vi "GeoData.vi"() -> ()   [LabVIEW 2017] (continued)
63130\t29189\tSaint louis\tMO\tSt. Louis County\tH1\n63133\t29189\tSaint louis\tMO\tSt. Louis County\tH1\n63138\t29189\tSaint louis\tMO\tSt. Louis County\tH1\n63011\t29189\tBallwin\tMO\tSt. Louis County\tH1\n63006\t29189\tChesterfield\tMO\tSt. Louis County\tH1\n63042\t29189\tHazelwood\tMO\tSt. Louis County\tH1\n63141\t29189\tSaint louis\tMO\tSt. Louis County\tH1\n63140\t29189\tSaint louis\tMO\tSt. Louis County\tH1\n63021\t29189\tBallwin\tMO\tSt. Louis County\tH1\n63117\t29189\tSaint louis\tMO\tSt. Louis County\tH1\n63121\t29189\tSaint louis\tMO\tSt. Louis County\tH1\n63126\t29189\tSaint louis\tMO\tSt. Louis County\tH1\n63025\t29189\tEureka\tMO\tSt. Louis County\tH1\n63022\t29189\tBallwin\tMO\tSt. Louis County\tH1\n63045\t29189\tEarth city\tMO\tSt. Louis County\tH1\n63167\t29189\tSaint louis\tMO\tSt. Louis County\tH1\n65340\t29195\tMarshall\tMO\tSaline County\tH1\n65349\t29195\tSlater\tMO\tSaline County\tH1\n64020\t29195\tConcordia\tMO\tSaline County\tH1\n65351\t29195\tSweet springs\tMO\tSaline County\tH1\n65339\t29195\tMalta bend\tMO\tSaline County\tH1\n65344\t29195\tMiami\tMO\tSaline County\tH1\n65322\t29195\tBlackwater\tMO\tSaline County\tH1\n65347\t29195\tNelson\tMO\tSaline County\tH1\n65320\t29195\tArrow rock\tMO\tSaline County\tH1\n65333\t29195\tHoustonia\tMO\tSaline County\tH1\n64096\t29195\tWaverly\tMO\tSaline County\tH1\n65330\t29195\tGilliam\tMO\tSaline County\tH1\n65327\t29195\tEmma\tMO\tSaline County\tH1\n65321\t29195\tBlackburn\tMO\tSaline County\tH1\n63535\t29197\tCoatsville\tMO\tSchuyler County\tH1\n63548\t29197\tLancaster\tMO\tSchuyler County\tH1\n63536\t29197\tDowning\tMO\tSchuyler County\tH1\n63541\t29197\tGlenwood\tMO\tSchuyler County\tH1\n63561\t29197\tQueen city\tMO\tSchuyler County\tH1\n63546\t29197\tGreentop\tMO\tSchuyler County\tH1\n63543\t29199\tGorin\tMO\tScotland County\tH1\n63555\t29199\tMemphis\tMO\tScotland County\tH1\n63563\t29199\tRutledge\tMO\tScotland County\tH1\n63442\t29199\tGranger\tMO\tScotland County\tH1\n63432\t29199\tArbela\tMO\tScotland County\tH1\n63735\t29201\tBell city\tMO\tScott County\tH1\n63742\t29201\tCommerce\tMO\tScott County\tH1\n63758\t29201\tKelso\tMO\tScott County\tH1\n63774\t29201\tPerkins\tMO\tScott County\tH1\n63771\t29201\tOran\tMO\tScott County\tH1\n63740\t29201\tChaffee\tMO\tScott County\tH1\n63834\t29201\tCharleston\tMO\tScott County\tH1\n63780\t29201\tScott city\tMO\tScott County\tH1\n63801\t29201\tSikeston\tMO\tScott County\tH1\n63823\t29201\tBertrand\tMO\tScott County\tH1\n63736\t29201\tBenton\tMO\tScott County\tH1\n63784\t29201\tVanduser\tMO\tScott County\tH1\n63767\t29201\tMorley\tMO\tScott County\tH1\n63824\t29201\tBlodgett\tMO\tScott County\tH1\n65438\t29203\tBirch tree\tMO\tShannon County\tH1\n65479\t29203\tHartshorn\tMO\tShannon County\tH1\n65571\t29203\tSummersville\tMO\tShannon County\tH1\n65588\t29203\tWinona\tMO\tShannon County\tH1\n65546\t29203\tMontier\tMO\tShannon County\tH1\n65560\t29203\tSalem\tMO\tShannon County\tH1\n65466\t29203\tEminence\tMO\tShannon County\tH1\n65548\t29203\tMountain view\tMO\tShannon County\tH1\n63450\t29205\tLentner\tMO\tShelby County\tH1\n63468\t29205\tShelbina\tMO\tShelby County\tH1\n63443\t29205\tHunnewell\tMO\tShelby County\tH1\n63434\t29205\tBethel\tMO\tShelby County\tH1\n63451\t29205\tLeonard\tMO\tShelby County\tH1\n63469\t29205\tShelbyville\tMO\tShelby County\tH1\n63437\t29205\tClarence\tMO\tShelby County\tH1\n63440\t29205\tEwing\tMO\tShelby County\tH1\n63439\t29205\tEmden\tMO\tShelby County\tH1\n63735\t29207\tBell city\tMO\tStoddard County\tH1\n63825\t29207\tBloomfield\tMO\tStoddard County\tH1\n63730\t29207\tAdvance\tMO\tStoddard County\tH1\n63850\t29207\tGrayridge\tMO\tStoddard County\tH1\n63771\t29207\tOran\tMO\tStoddard County\tH1\n63822\t29207\tBernie\tMO\tStoddard County\tH1\n63936\t29207\tDudley\tMO\tStoddard County\tH1\n63833\t29207\tCatron\tMO\tStoddard County\tH1\n63846\t29207\tEssex\tMO\tStoddard County\tH1\n63801\t29207\tSikeston\tMO\tStoddard County\tH1\n63870\t29207\tParma\tMO\tStoddard County\tH1\n63738\t29207\tBrownwood\tMO\tStoddard County\tH1\n63960\t29207\tPuxico\tMO\tStoddard County\tH1\n63841\t29207\tDexter\tMO\tStoddard County\tH1\n65714\t29209\tNixa\tMO\tStone County\tH1\n65656\t29209\tGalena\tMO\tStone County\tH1\n65633\t29209\tCrane\tMO\tStone County\tH1\n65616\t29209\tBranson\tMO\tStone County\tH1\n65705\t29209\tMarionville\tMO\tStone County\tH1\n65669\t29209\tHighlandville\tMO\tStone County\tH1\n65728\t29209\tPonce de leon\tMO\tStone County\tH1\n65624\t29209\tCape fair\tMO\tStone County\tH1\n65610\t29209\tBillings\tMO\tStone County\tH1\n65611\t29209\tBlue eye\tMO\tStone County\tH1\n65681\t29209\tLampe\tMO\tStone County\tH1\n65675\t29209\tHurley\tMO\tStone County\tH1\n65605\t29209\tAurora\tMO\tStone County\tH1\n65737\t29209\tReeds spring\tMO\tStone County\tH1\n65631\t29209\tClever\tMO\tStone County\tH1\n65747\t29209\tShell knob\tMO\tStone County\tH1\n65754\t29209\tSpokane\tMO\tStone County\tH1\n65686\t29209\tKimberling city\tMO\tStone County\tH1\n64641\t29211\tGalt\tMO\tSullivan County\tH1\n63556\t29211\tMilan\tMO\tSullivan County\tH1\n63560\t29211\tPollock\tMO\tSullivan County\tH1\n63566\t29211\tWinigan\tMO\tSullivan County\tH1\n63565\t29211\tUnionville\tMO\tSullivan County\tH1\n63557\t29211\tNew boston\tMO\tSullivan County\tH1\n63545\t29211\tGreen city\tMO\tSullivan County\tH1\n64652\t29211\tLaredo\tMO\tSullivan County\tH1\n64646\t29211\tHumphreys\tMO\tSullivan County\tH1\n64667\t29211\tNewtown\tMO\tSullivan County\tH1\n63544\t29211\tGreen castle\tMO\tSullivan County\tH1\n64630\t29211\tBrowning\tMO\tSullivan County\tH1\n64645\t29211\tHarris\tMO\tSullivan County\tH1\n65615\t29213\tBranson\tMO\tTaney County\tH1\n65739\t29213\tRidgedale\tMO\tTaney County\tH1\n65761\t29213\tTheodosia\tMO\tTaney County\tH1\n65614\t29213\tBradleyville\tMO\tTaney County\tH1\n65616\t29213\tBranson\tMO\tTaney County\tH1\n65740\t29213\tRockaway beach\tMO\tTaney County\tH1\n65627\t29213\tCedarcreek\tMO\tTaney County\tH1\n65759\t29213\tTaneyville\tMO\tTaney County\tH1\n65771\t29213\tWalnut shade\tMO\tTaney County\tH1\n65731\t29213\tPowersite\tMO\tTaney County\tH1\n65611\t29213\tBlue eye\tMO\tTaney County\tH1\n65679\t29213\tKirbyville\tMO\tTaney County\tH1\n65726\t29213\tPoint lookout\tMO\tTaney County\tH1\n65673\t29213\tHollister\tMO\tTaney County\tH1\n65608\t29213\tAva\tMO\tTaney County\tH1\n65680\t29213\tKissee mills\tMO\tTaney County\tH1\n65653\t29213\tForsyth\tMO\tTaney County\tH1\n65733\t29213\tProtem\tMO\tTaney County\tH1\n65737\t29213\tReeds spring\tMO\tTaney County\tH1\n65672\t29213\tHollister\tMO\tTaney County\tH1\n65744\t29213\tRueter\tMO\tTaney County\tH1\n65630\t29213\tChestnutridge\tMO\tTaney County\tH1\n65793\t29215\tWillow springs\tMO\tTexas County\tH1\n65564\t29215\tSolo\tMO\tTexas County\tH1\n65470\t29215\tFalcon\tMO\tTexas County\tH1\n65484\t29215\tHuggins\tMO\tTexas County\tH1\n65589\t29215\tYukon\tMO\tTexas County\tH1\n65557\t29215\tRoby\tMO\tTexas County\tH1\n65689\t29215\tCabool\tMO\tTexas County\tH1\n65711\t29215\tMountain grove\tMO\tTexas County\tH1\n65468\t29215\tEunice\tMO\tTexas County\tH1\n65552\t29215\tPlato\tMO\tTexas County\tH1\n65660\t29215\tGraff\tMO\tTexas County\tH1\n65483\t29215\tHouston\tMO\tTexas County\tH1\n65479\t29215\tHartshorn\tMO\tTexas County\tH1\n65571\t29215\tSummersville\tMO\tTexas County\tH1\n65555\t29215\tRaymondville\tMO\tTexas County\tH1\n65436\t29215\tBeulah\tMO\tTexas County\tH1\n65560\t29215\tSalem\tMO\tTexas County\tH1\n65542\t29215\tLicking\tMO\tTexas County\tH1\n65570\t29215\tSuccess\tMO\tTexas County\tH1\n65548\t29215\tMountain view\tMO\tTexas County\tH1\n65464\t29215\tElk creek\tMO\tTexas County\tH1\n65444\t29215\tBucyrus\tMO\tTexas County\tH1\n64767\t29217\tMilo\tMO\tVernon County\tH1\n64728\t29217\tBronaugh\tMO\tVernon County\tH1\n64772\t29217\tNevada\tMO\tVernon County\tH1\n64741\t29217\tDeerfield\tMO\tVernon County\tH1\n64783\t29217\tSchell city\tMO\tVernon County\tH1\n64765\t29217\tMetz\tMO\tVernon County\tH1\n64744\t29217\tEl dorado springs\tMO\tVernon County\tH1\n64752\t29217\tHume\tMO\tVernon County\tH1\n64750\t29217\tHarwood\tMO\tVernon County\tH1\n64779\t29217\tRich hill\tMO\tVernon County\tH1\n64778\t29217\tRichards\tMO\tVernon County\tH1\n64784\t29217\tSheldon\tMO\tVernon County\tH1\n64771\t29217\tMoundville\tMO\tVernon County\tH1\n64790\t29217\tWalker\tMO\tVernon County\tH1\n63381\t29219\tTruxton\tMO\tWarren County\tH1\n63351\t29219\tJonesburg\tMO\tWarren County\tH1\n63363\t29219\tNew florence\tMO\tWarren County\tH1\n63380\t29219\tTruesdale\tMO\tWarren County\tH1\n63390\t29219\tWright city\tMO\tWarren County\tH1\n63348\t29219\tForistell\tMO\tWarren County\tH1\n63378\t29219\tTreloar\tMO\tWarren County\tH1\n63379\t29219\tTroy\tMO\tWarren County\tH1\n63383\t29219\tWarrenton\tMO\tWarren County\tH1\n65041\t29219\tHermann\tMO\tWarren County\tH1\n63357\t29219\tMarthasville\tMO\tWarren County\tH1\n63349\t29219\tHawk point\tMO\tWarren County\tH1\n63342\t29219\tDutzow\tMO\tWarren County\tH1\n63624\t29221\tBismarck\tMO\tWashington County\tH1\n63648\t29221\tIrondale\tMO\tWashington County\tH1\n65441\t29221\tBourbon\tMO\tWashington County\tH1\n63622\t29221\tBelgrade\tMO\tWashington County\tH1\n63628\t29221\tBonne terre\tMO\tWashington County\tH1\n63080\t29221\tSullivan\tMO\tWashington County\tH1\n63630\t29221\tCadet\tMO\tWashington County\tH1\n65565\t29221\tSteelville\tMO\tWashington County\tH1\n63023\t29221\tDittmer\tMO\tWashington County\tH1\n63020\t29221\tDe soto\tMO\tWashington County\tH1\n63071\t29221\tRichwoods\tMO\tWashington County\tH1\n63060\t29221\tLonedell\tMO\tWashington County\tH1\n63660\t29221\tMineral point\tMO\tWashington County\tH1\n63626\t29221\tBlackwell\tMO\tWashington County\tH1\n63664\t29221\tPotosi\tMO\tWashington County\tH1\n63030\t29221\tFletcher\tMO\tWashington County\tH1\n63631\t29221\tCaledonia\tMO\tWashington County\tH1\n63674\t29221\tTiff\tMO\tWashington County\tH1\n63638\t29223\tEllington\tMO\tWayne County\tH1\n63763\t29223\tMc gee\tMO\tWayne County\tH1\n63950\t29223\tLodi\tMO\tWayne County\tH1\n63957\t29223\tPiedmont\tMO\tWayne County\tH1\n63966\t29223\tWappapello\tMO\tWayne County\tH1\n63934\t29223\tClubb\tMO\tWayne County\tH1\n63952\t29223\tMill spring\tMO\tWayne County\tH1\n63956\t29223\tPatterson\tMO\tWayne County\tH1\n63967\t29223\tWilliamsville\tMO\tWayne County\tH1\n63964\t29223\tSilva\tMO\tWayne County\tH1\n63944\t29223\tGreenville\tMO\tWayne County\tH1\n63960\t29223\tPuxico\tMO\tWayne County\tH1\n63951\t29223\tLowndes\tMO\tWayne County\tH1\n65706\t29225\tMarshfield\tMO\tWebster County\tH1\n65713\t29225\tNiangua\tMO\tWebster County\tH1\n65632\t29225\tConway\tMO\tWebster County\tH1\n65667\t29225\tHartville\tMO\tWebster County\tH1\n65644\t29225\tElkland\tMO\tWebster County\tH1\n65662\t29225\tGrovespring\tMO\tWebster County\tH1\n65746\t29225\tSeymour\tMO\tWebster County\tH1\n65757\t29225\tStrafford\tMO\tWebster County\tH1\n65648\t29225\tFair grove\tMO\tWebster County\tH1\n65652\t29225\tFordland\tMO\tWebster County\tH1\n65742\t29225\tRogersville\tMO\tWebster County\tH1\n65636\t29225\tDiggins\tMO\tWebster County\tH1\n64486\t29227\tSheridan\tMO\tWorth County\tH1\n64441\t29227\tDenver\tMO\tWorth County\tH1\n64456\t29227\tGrant city\tMO\tWorth County\tH1\n64420\t29227\tAllendale\tMO\tWorth County\tH1\n64499\t29227\tWorth\tMO\tWorth County\tH1\n65470\t29229\tFalcon\tMO\tWright County\tH1\n65706\t29229\tMarshfield\tMO\tWright County\tH1\n65713\t29229\tNiangua\tMO\tWright County\tH1\n65667\t29229\tHartville\tMO\tWright County\tH1\n65543\t29229\tLynchburg\tMO\tWright County\tH1\n65711\t29229\tMountain grove\tMO\tWright County\tH1\n65704\t29229\tMansfield\tMO\tWright County\tH1\n65662\t29229\tGrovespring\tMO\tWright County\tH1\n65660\t29229\tGraff\tMO\tWright County\tH1\n65746\t29229\tSeymour\tMO\tWright County\tH1\n65717\t29229\tNorwood\tMO\tWright County\tH1\n65702\t29229\tMacomb\tMO\tWright County\tH1\n63105\t29510\tSaint louis\tMO\tSt. Louis city\tC7\n63107\t29510\tSaint louis\tMO\tSt. Louis city\tC7\n63119\t29510\tSaint louis\tMO\tSt. Louis city\tC7\n63166\t29510\tSaint louis\tMO\tSt. Louis city\tC7\n63123\t29510\tSaint louis\tMO\tSt. Louis city\tC7\n63103\t29510\tSaint louis\tMO\tSt. Louis city\tC7\n63136\t29510\tSaint louis\tMO\tSt. Louis city\tC7\n63139\t29510\tSaint louis\tMO\tSt. Louis city\tC7\n63137\t29510\tSaint louis\tMO\tSt. Louis city\tC7\n63112\t29510\tSaint louis\tMO\tSt. Louis city\tC7\n63102\t29510\tSaint louis\tMO\tSt. Louis city\tC7\n63118\t29510\tSaint louis\tMO\tSt. Louis city\tC7\n63101\t29510\tSaint louis\tMO\tSt. Louis city\tC7\n63180\t29510\tSaint louis\tMO\tSt. Louis city\tC7\n63104\t29510\tSaint louis\tMO\tSt. Louis city\tC7\n63116\t29510\tSaint louis\tMO\tSt. Louis city\tC7\n63120\t29510\tSaint louis\tMO\tSt. Louis city\tC7\n63143\t29510\tSaint louis\tMO\tSt. Louis city\tC7\n63147\t29510\tSaint louis\tMO\tSt. Louis city\tC7\n63125\t29510\tSaint louis\tMO\tSt. Louis city\tC7\n63160\t29510\tSaint louis\tMO\tSt. Louis city\tC7\n63106\t29510\tSaint louis\tMO\tSt. Louis city\tC7\n63108\t29510\tSaint louis\tMO\tSt. Louis city\tC7\n63156\t29510\tSaint louis\tMO\tSt. Louis city\tC7\n63115\t29510\tSaint louis\tMO\tSt. Louis city\tC7\n63111\t29510\tSaint louis\tMO\tSt. Louis city\tC7\n63113\t29510\tSaint louis\tMO\tSt. Louis city\tC7\n63130\t29510\tSaint louis\tMO\tSt. Louis city\tC7\n63133\t29510\tSaint louis\tMO\tSt. Louis city\tC7\n63138\t29510\tSaint louis\tMO\tSt. Louis city\tC7\n63164\t29510\tSaint louis\tMO\tSt. Louis city\tC7\n63109\t29510\tSaint louis\tMO\tSt. Louis city\tC7\n63178\t29510\tSaint louis\tMO\tSt. Louis city\tC7\n63110\t29510\tSaint louis\tMO\tSt. Louis city\tC7\n63117\t29510\tSaint louis\tMO\tSt. Louis city\tC7\n63155\t29510\tSaint louis\tMO\tSt. Louis city\tC7\n63177\t29510\tSaint louis\tMO\tSt. Louis city\tC7\n63150\t29510\tSaint louis\tMO\tSt. Louis city\tC7\n59739\t30001\tLima\tMT\tBeaverhead County\tH1\n59746\t30001\tPolaris\tMT\tBeaverhead County\tH1\n59761\t30001\tWisdom\tMT\tBeaverhead County\tH1\n59724\t30001\tDell\tMT\tBeaverhead County\tH1\n59725\t30001\tDillon\tMT\tBeaverhead County\tH1\n59762\t30001\tWise river\tMT\tBeaverhead County\tH1\n59732\t30001\tGlen\tMT\tBeaverhead County\tH1\n59736\t30001\tJackson\tMT\tBeaverhead County\tH1\n59727\t30001\tDivide\tMT\tBeaverhead County\tH1\n59101\t30003\tBillings\tMT\tBig Horn County\tH1\n59034\t30003\tHardin\tMT\tBig Horn County\tH1\n59016\t30003\tBusby\tMT\tBig Horn County\tH1\n59025\t30003\tDecker\tMT\tBig Horn County\tH1\n59064\t30003\tPompeys pillar\tMT\tBig Horn County\tH1\n59066\t30003\tPryor\tMT\tBig Horn County\tH1\n59050\t30003\tLodge grass\tMT\tBig Horn County\tH1\n59022\t30003\tCrow agency\tMT\tBig Horn County\tH1\n59075\t30003\tSaint xavier\tMT\tBig Horn County\tH1\n59024\t30003\tCuster\tMT\tBig Horn County\tH1\n59089\t30003\tWyola\tMT\tBig Horn County\tH1\n59031\t30003\tGarryowen\tMT\tBig Horn County\tH1\n59035\t30003\tFort smith\tMT\tBig Horn County\tH1\n59526\t30005\tHarlem\tMT\tBlaine County\tH1\n59520\t30005\tBig sandy\tMT\tBlaine County\tH1\n59523\t30005\tChinook\tMT\tBlaine County\tH1\n59529\t30005\tHogeland\tMT\tBlaine County\tH1\n59547\t30005\tZurich\tMT\tBlaine County\tH1\n59535\t30005\tLloyd\tMT\tBlaine County\tH1\n59501\t30005\tHavre\tMT\tBlaine County\tH1\n59542\t30005\tTurner\tMT\tBlaine County\tH1\n59527\t30005\tHays\tMT\tBlaine County\tH1\n59524\t30005\tDodson\tMT\tBlaine County\tH1\n59635\t30007\tEast helena\tMT\tBroadwater County\tH1\n59721\t30007\tCardwell\tMT\tBroadwater County\tH1\n59641\t30007\tRadersburg\tMT\tBroadwater County\tH1\n59644\t30007\tTownsend\tMT\tBroadwater County\tH1\n59647\t30007\tWinston\tMT\tBroadwater County\tH1\n59643\t30007\tToston\tMT\tBroadwater County\tH1\n59645\t30007\tWhite sulphur springs\tMT\tBroadwater County\tH1\n59752\t30007\tThree forks\tMT\tBroadwater County\tH1\n59008\t30009\tBelfry\tMT\tCarbon County\tH1\n59044\t30009\tLaurel\tMT\tCarbon County\tH1\n59068\t30009\tRed lodge\tMT\tCarbon County\tH1\n59014\t30009\tBridger\tMT\tCarbon County\tH1\n59071\t30009\tRoscoe\tMT\tCarbon County\tH1\n59041\t30009\tJoliet\tMT\tCarbon County\tH1\n59029\t30009\tFromberg\tMT\tCarbon County\tH1\n59019\t30009\tColumbus\tMT\tCarbon County\tH1\n59001\t30009\tAbsarokee\tMT\tCarbon County\tH1\n59026\t30009\tEdgar\tMT\tCarbon County\tH1\n59070\t30009\tRoberts\tMT\tCarbon County\tH1\n59013\t30009\tBoyd\tMT\tCarbon County\tH1\n59007\t30009\tBearcreek\tMT\tCarbon County\tH1\n59311\t30011\tAlzada\tMT\tCarter County\tH1\n59319\t30011\tCapitol\tMT\tCarter County\tH1\n59332\t30011\tHammond\tMT\tCarter County\tH1\n59324\t30011\tEkalaka\tMT\tCarter County\tH1\n59316\t30011\tBoyes\tMT\tCarter County\tH1\n59405\t30013\tGreat falls\tMT\tCascade County\tH1\n59401\t30013\tGreat falls\tMT\tCascade County\tH1\n59468\t30013\tPower\tMT\tCascade County\tH1\n59412\t30013\tBelt\tMT\tCascade County\tH1\n59440\t30013\tFloweree\tMT\tCascade County\tH1\n59472\t30013\tSand coulee\tMT\tCascade County\tH1\n59414\t30013\tBlack eagle\tMT\tCascade County\tH1\n59483\t30013\tSun river\tMT\tCascade County\tH1\n59487\t30013\tVaughn\tMT\tCascade County\tH1\n59436\t30013\tFairfield\tMT\tCascade County\tH1\n59443\t30013\tFort shaw\tMT\tCascade County\tH1\n59477\t30013\tSimms\tMT\tCascade County\tH1\n59403\t30013\tGreat falls\tMT\tCascade County\tH1\n59465\t30013\tNeihart\tMT\tCascade County\tH1\n59485\t30013\tUlm\tMT\tCascade County\tH1\n59404\t30013\tGreat falls\tMT\tCascade County\tH1\n59402\t30013\tMalmstrom afb\tMT\tCascade County\tH1\n59480\t30013\tStockett\tMT\tCascade County\tH1\n59421\t30013\tCascade\tMT\tCascade County\tH1\n59406\t30013\tGreat falls\tMT\tCascade County\tH1\n59463\t30013\tMonarch\tMT\tCascade County\tH1\n59460\t30015\tLoma\tMT\tChouteau County\tH1\n59520\t30015\tBig sandy\tMT\tChouteau County\tH1\n59442\t30015\tFort benton\tMT\tChouteau County\tH1\n59447\t30015\tGeyser\tMT\tChouteau County\tH1\n59412\t30015\tBelt\tMT\tChouteau County\tH1\n59440\t30015\tFloweree\tMT\tChouteau County\tH1\n59540\t30015\tRudyard\tMT\tChouteau County\tH1\n59433\t30015\tDutton\tMT\tChouteau County\tH1\n59420\t30015\tCarter\tMT\tChouteau County\tH1\n59416\t30015\tBrady\tMT\tChouteau County\tH1\n59450\t30015\tHighwood\tMT\tChouteau County\tH1\n59404\t30015\tGreat falls\tMT\tChouteau County\tH1\n59446\t30015\tGeraldine\tMT\tChouteau County\tH1\n59521\t30015\tBox elder\tMT\tChouteau County\tH1\n59301\t30017\tMiles city\tMT\tCuster County\tH1\n59349\t30017\tTerry\tMT\tCuster County\tH1\n59336\t30017\tIsmay\tMT\tCuster County\tH1\n59338\t30017\tKinsey\tMT\tCuster County\tH1\n59351\t30017\tVolborg\tMT\tCuster County\tH1\n59253\t30019\tPeerless\tMT\tDaniels County\tH1\n59201\t30019\tWolf point\tMT\tDaniels County\tH1\n59263\t30019\tScobey\tMT\tDaniels County\tH1\n59222\t30019\tFlaxville\tMT\tDaniels County\tH1\n59260\t30019\tRichland\tMT\tDaniels County\tH1\n59276\t30019\tWhitetail\tMT\tDaniels County\tH1\n59257\t30019\tRedstone\tMT\tDaniels County\tH1\n59339\t30021\tLindsay\tMT\tDawson County\tH1\n59315\t30021\tBloomfield\tMT\tDawson County\tH1\n59259\t30021\tRichey\tMT\tDawson County\tH1\n59330\t30021\tGlendive\tMT\tDawson County\tH1\n59353\t30021\tWibaux\tMT\tDawson County\tH1\n59262\t30021\tSavage\tMT\tDawson County\tH1\n59215\t30021\tCircle\tMT\tDawson County\tH1\n59701\t30023\tButte\tMT\tDeer Lodge County\tH6\n59711\t30023\tAnaconda\tMT\tDeer Lodge County\tH6\n59762\t30023\tWise river\tMT\tDeer Lodge County\tH6\n59756\t30023\tWarm springs\tMT\tDeer Lodge County\tH6\n59722\t30023\tDeer lodge\tMT\tDeer Lodge County\tH6\n59344\t30025\tPlevna\tMT\tFallon County\tH1\n59354\t30025\tWillard\tMT\tFallon County\tH1\n59313\t30025\tBaker\tMT\tFallon County\tH1\n59336\t30025\tIsmay\tMT\tFallon County\tH1\n59462\t30027\tMoccasin\tMT\tFergus County\tH1\n59457\t30027\tLewistown\tMT\tFergus County\tH1\n59441\t30027\tForest grove\tMT\tFergus County\tH1\n59489\t30027\tWinifred\tMT\tFergus County\tH1\n59430\t30027\tDenton\tMT\tFergus County\tH1\n59451\t30027\tHilger\tMT\tFergus County\tH1\n59424\t30027\tCoffee creek\tMT\tFergus County\tH1\n59464\t30027\tMoore\tMT\tFergus County\tH1\n59453\t30027\tJudith gap\tMT\tFergus County\tH1\n59087\t30027\tWinnett\tMT\tFergus County\tH1\n59032\t30027\tGrass range\tMT\tFergus County\tH1\n59418\t30027\tBuffalo\tMT\tFergus County\tH1\n59471\t30027\tRoy\tMT\tFergus County\tH1\n59917\t30029\tEureka\tMT\tFlathead County\tH1\n59928\t30029\tPolebridge\tMT\tFlathead County\tH1\n59916\t30029\tEssex\tMT\tFlathead County\tH1\n59921\t30029\tLake mc donald\tMT\tFlathead County\tH1\n59937\t30029\tWhitefish\tMT\tFlathead County\tH1\n59927\t30029\tOlney\tMT\tFlathead County\tH1\n59845\t30029\tHot springs\tMT\tFlathead County\tH1\n59912\t30029\tColumbia falls\tMT\tFlathead County\tH1\n59922\t30029\tLakeside\tMT\tFlathead County\tH1\n59932\t30029\tSomers\tMT\tFlathead County\tH1\n59913\t30029\tCoram\tMT\tFlathead County\tH1\n59925\t30029\tMarion\tMT\tFlathead County\tH1\n59903\t30029\tKalispell\tMT\tFlathead County\tH1\n59926\t30029\tMartin city\tMT\tFlathead County\tH1\n59936\t30029\tWest glacier\tMT\tFlathead County\tH1\n59901\t30029\tKalispell\tMT\tFlathead County\tH1\n59904\t30029\tKalispell\tMT\tFlathead County\tH1\n59911\t30029\tBigfork\tMT\tFlathead County\tH1\n59920\t30029\tKila\tMT\tFlathead County\tH1\n59919\t30029\tHungry horse\tMT\tFlathead County\tH1\n59086\t30031\tWilsall\tMT\tGallatin County\tH1\n59771\t30031\tBozeman\tMT\tGallatin County\tH1\n59721\t30031\tCardwell\tMT\tGallatin County\tH1\n59714\t30031\tBelgrade\tMT\tGallatin County\tH1\n59717\t30031\tBozeman\tMT\tGallatin County\tH1\n59716\t30031\tBig sky\tMT\tGallatin County\tH1\n59772\t30031\tBozeman\tMT\tGallatin County\tH1\n59715\t30031\tBozeman\tMT\tGallatin County\tH1\n59730\t30031\tGallatin gateway\tMT\tGallatin County\tH1\n59719\t30031\tBozeman\tMT\tGallatin County\tH1\n59760\t30031\tWillow creek\tMT\tGallatin County\tH1\n59758\t30031\tWest yellowstone\tMT\tGallatin County\tH1\n59741\t30031\tManhattan\tMT\tGallatin County\tH1\n59718\t30031\tBozeman\tMT\tGallatin County\tH1\n59752\t30031\tThree forks\tMT\tGallatin County\tH1\n59337\t30033\tJordan\tMT\tGarfield County\tH1\n59318\t30033\tBrusett\tMT\tGarfield County\tH1\n59322\t30033\tCohagen\tMT\tGarfield County\tH1\n59077\t30033\tSand springs\tMT\tGarfield County\tH1\n59058\t30033\tMosby\tMT\tGarfield County\tH1\n59417\t30035\tBrowning\tMT\tGlacier County\tH1\n59427\t30035\tCut bank\tMT\tGlacier County\tH1\n59434\t30035\tEast glacier park\tMT\tGlacier County\tH1\n59486\t30035\tValier\tMT\tGlacier County\tH1\n59411\t30035\tBabb\tMT\tGlacier County\tH1\n59072\t30037\tRoundup\tMT\tGolden Valley County\tH1\n59078\t30037\tShawmut\tMT\tGolden Valley County\tH1\n59074\t30037\tRyegate\tMT\tGolden Valley County\tH1\n59046\t30037\tLavina\tMT\tGolden Valley County\tH1\n59858\t30039\tPhilipsburg\tMT\tGranite County\tH1\n59711\t30039\tAnaconda\tMT\tGranite County\tH1\n59837\t30039\tHall\tMT\tGranite County\tH1\n59825\t30039\tClinton\tMT\tGranite County\tH1\n59832\t30039\tDrummond\tMT\tGranite County\tH1\n59520\t30041\tBig sandy\tMT\tHill County\tH1\n59523\t30041\tChinook\tMT\tHill County\tH1\n59530\t30041\tInverness\tMT\tHill County\tH1\n59532\t30041\tKremlin\tMT\tHill County\tH1\n59540\t30041\tRudyard\tMT\tHill County\tH1\n59501\t30041\tHavre\tMT\tHill County\tH1\n59528\t30041\tHingham\tMT\tHill County\tH1\n59521\t30041\tBox elder\tMT\tHill County\tH1\n59525\t30041\tGildford\tMT\tHill County\tH1\n59635\t30043\tEast helena\tMT\tJefferson County\tH1\n59721\t30043\tCardwell\tMT\tJefferson County\tH1\n59701\t30043\tButte\tMT\tJefferson County\tH1\n59632\t30043\tBoulder\tMT\tJefferson County\tH1\n59759\t30043\tWhitehall\tMT\tJefferson County\tH1\n59601\t30043\tHelena\tMT\tJefferson County\tH1\n59631\t30043\tBasin\tMT\tJefferson County\tH1\n59634\t30043\tClancy\tMT\tJefferson County\tH1\n59638\t30043\tJefferson city\tMT\tJefferson County\tH1\n59752\t30043\tThree forks\tMT\tJefferson County\tH1\n59462\t30045\tMoccasin\tMT\tJudith Basin County\tH1\n59469\t30045\tRaynesford\tMT\tJudith Basin County\tH1\n59447\t30045\tGeyser\tMT\tJudith Basin County\tH1\n59452\t30045\tHobson\tMT\tJudith Basin County\tH1\n59430\t30045\tDenton\tMT\tJudith Basin County\tH1\n59479\t30045\tStanford\tMT\tJudith Basin County\tH1\n59424\t30045\tCoffee creek\tMT\tJudith Basin County\tH1\n59464\t30045\tMoore\tMT\tJudith Basin County\tH1\n59418\t30045\tBuffalo\tMT\tJudith Basin County\tH1\n59931\t30047\tRollins\tMT\tLake County\tH1\n59855\t30047\tPablo\tMT\tLake County\tH1\n59821\t30047\tArlee\tMT\tLake County\tH1\n59915\t30047\tElmo\tMT\tLake County\tH1\n59845\t30047\tHot springs\tMT\tLake County\tH1\n59922\t30047\tLakeside\tMT\tLake County\tH1\n59865\t30047\tSaint ignatius\tMT\tLake County\tH1\n59929\t30047\tProctor\tMT\tLake County\tH1\n59824\t30047\tCharlo\tMT\tLake County\tH1\n59860\t30047\tPolson\tMT\tLake County\tH1\n59910\t30047\tBig arm\tMT\tLake County\tH1\n59864\t30047\tRonan\tMT\tLake County\tH1\n59863\t30047\tRavalli\tMT\tLake County\tH1\n59914\t30047\tDayton\tMT\tLake County\tH1\n59911\t30047\tBigfork\tMT\tLake County\tH1\n59635\t30049\tEast helena\tMT\tLewis and Clark County\tH1\n59626\t30049\tHelena\tMT\tLewis and Clark County\tH1\n59623\t30049\tHelena\tMT\tLewis and Clark County\tH1\n59648\t30049\tWolf creek\tMT\tLewis and Clark County\tH1\n59636\t30049\tFort harrison\tMT\tLewis and Clark County\tH1\n59620\t30049\tHelena\tMT\tLewis and Clark County\tH1\n59604\t30049\tHelena\tMT\tLewis and Clark County\tH1\n59640\t30049\tMarysville\tMT\tLewis and Clark County\tH1\n59639\t30049\tLincoln\tMT\tLewis and Clark County\tH1\n59624\t30049\tHelena\tMT\tLewis and Clark County\tH1\n59410\t30049\tAugusta\tMT\tLewis and Clark County\tH1\n59602\t30049\tHelena\tMT\tLewis and Clark County\tH1\n59601\t30049\tHelena\tMT\tLewis and Clark County\tH1\n59634\t30049\tClancy\tMT\tLewis and Clark County\tH1\n59421\t30049\tCascade\tMT\tLewis and Clark County\tH1\n59625\t30049\tHelena\tMT\tLewis and Clark County\tH1\n59633\t30049\tCanyon creek\tMT\tLewis and Clark County\tH1\n59545\t30051\tWhitlash\tMT\tLiberty County\tH1\n59522\t30051\tChester\tMT\tLiberty County\tH1\n59456\t30051\tLedger\tMT\tLiberty County\tH1\n59444\t30051\tGalata\tMT\tLiberty County\tH1\n59531\t30051\tJoplin\tMT\tLiberty County\tH1\n59461\t30051\tLothair\tMT\tLiberty County\tH1\n59917\t30053\tEureka\tMT\tLincoln County\tH1\n59930\t30053\tRexford\tMT\tLincoln County\tH1\n59935\t30053\tTroy\tMT\tLincoln County\tH1\n59918\t30053\tFortine\tMT\tLincoln County\tH1\n59925\t30053\tMarion\tMT\tLincoln County\tH1\n59934\t30053\tTrego\tMT\tLincoln County\tH1\n59933\t30053\tStryker\tMT\tLincoln County\tH1\n59923\t30053\tLibby\tMT\tLincoln County\tH1\n59315\t30055\tBloomfield\tMT\tMcCone County\tH1\n59259\t30055\tRichey\tMT\tMcCone County\tH1\n59274\t30055\tVida\tMT\tMcCone County\tH1\n59223\t30055\tFort peck\tMT\tMcCone County\tH1\n59201\t30055\tWolf point\tMT\tMcCone County\tH1\n59214\t30055\tBrockway\tMT\tMcCone County\tH1\n59215\t30055\tCircle\tMT\tMcCone County\tH1\n59721\t30057\tCardwell\tMT\tMadison County\tH1\n59735\t30057\tHarrison\tMT\tMadison County\tH1\n59754\t30057\tTwin bridges\tMT\tMadison County\tH1\n59729\t30057\tEnnis\tMT\tMadison County\tH1\n59747\t30057\tPony\tMT\tMadison County\tH1\n59749\t30057\tSheridan\tMT\tMadison County\tH1\n59755\t30057\tVirginia city\tMT\tMadison County\tH1\n59759\t30057\tWhitehall\tMT\tMadison County\tH1\n59741\t30057\tManhattan\tMT\tMadison County\tH1\n59740\t30057\tMc allister\tMT\tMadison County\tH1\n59720\t30057\tCameron\tMT\tMadison County\tH1\n59751\t30057\tSilver star\tMT\tMadison County\tH1\n59718\t30057\tBozeman\tMT\tMadison County\tH1\n59710\t30057\tAlder\tMT\tMadison County\tH1\n59745\t30057\tNorris\tMT\tMadison County\tH1\n59086\t30059\tWilsall\tMT\tMeagher County\tH1\n59642\t30059\tRingling\tMT\tMeagher County\tH1\n59053\t30059\tMartinsdale\tMT\tMeagher County\tH1\n59645\t30059\tWhite sulphur springs\tMT\tMeagher County\tH1\n59830\t30061\tDe borgia\tMT\tMineral County\tH1\n59872\t30061\tSuperior\tMT\tMineral County\tH1\n59820\t30061\tAlberton\tMT\tMineral County\tH1\n59859\t30061\tPlains\tMT\tMineral County\tH1\n59867\t30061\tSaltese\tMT\tMineral County\tH1\n59866\t30061\tSaint regis\tMT\tMineral County\tH1\n59801\t30063\tMissoula\tMT\tMissoula County\tH1\n59823\t30063\tBonner\tMT\tMissoula County\tH1\n59826\t30063\tCondon\tMT\tMissoula County\tH1\n59833\t30063\tFlorence\tMT\tMissoula County\tH1\n59802\t30063\tMissoula\tMT\tMissoula County\tH1\n59804\t30063\tMissoula\tMT\tMissoula County\tH1\n59834\t30063\tFrenchtown\tMT\tMissoula County\tH1\n59868\t30063\tSeeley lake\tMT\tMissoula County\tH1\n59851\t30063\tMilltown\tMT\tMissoula County\tH1\n59847\t30063\tLolo\tMT\tMissoula County\tH1\n59821\t30063\tArlee\tMT\tMissoula County\tH1\n59808\t30063\tMissoula\tMT\tMissoula County\tH1\n59806\t30063\tMissoula\tMT\tMissoula County\tH1\n59807\t30063\tMissoula\tMT\tMissoula County\tH1\n59825\t30063\tClinton\tMT\tMissoula County\tH1\n59803\t30063\tMissoula\tMT\tMissoula County\tH1\n59812\t30063\tMissoula\tMT\tMissoula County\tH1\n59846\t30063\tHuson\tMT\tMissoula County\tH1\n59820\t30063\tAlberton\tMT\tMissoula County\tH1\n59072\t30065\tRoundup\tMT\tMusselshell County\tH1\n59046\t30065\tLavina\tMT\tMusselshell County\tH1\n59059\t30065\tMusselshell\tMT\tMusselshell County\tH1\n59054\t30065\tMelstone\tMT\tMusselshell County\tH1\n59015\t30065\tBroadview\tMT\tMusselshell County\tH1\n59047\t30067\tLivingston\tMT\tPark County\tH1\n59086\t30067\tWilsall\tMT\tPark County\tH1\n59081\t30067\tSilver gate\tMT\tPark County\tH1\n59020\t30067\tCooke city\tMT\tPark County\tH1\n59027\t30067\tEmigrant\tMT\tPark County\tH1\n59030\t30067\tGardiner\tMT\tPark County\tH1\n59715\t30067\tBozeman\tMT\tPark County\tH1\n59018\t30067\tClyde park\tMT\tPark County\tH1\n59052\t30067\tMc leod\tMT\tPark County\tH1\n59082\t30067\tSpringdale\tMT\tPark County\tH1\n59065\t30067\tPray\tMT\tPark County\tH1\n59084\t30069\tTeigen\tMT\tPetroleum County\tH1\n59087\t30069\tWinnett\tMT\tPetroleum County\tH1\n59058\t30069\tMosby\tMT\tPetroleum County\tH1\n59538\t30071\tMalta\tMT\tPhillips County\tH1\n59546\t30071\tZortman\tMT\tPhillips County\tH1\n59261\t30071\tSaco\tMT\tPhillips County\tH1\n59524\t30071\tDodson\tMT\tPhillips County\tH1\n59241\t30071\tHinsdale\tMT\tPhillips County\tH1\n59537\t30071\tLoring\tMT\tPhillips County\tH1\n59544\t30071\tWhitewater\tMT\tPhillips County\tH1\n59425\t30073\tConrad\tMT\tPondera County\tH1\n59456\t30073\tLedger\tMT\tPondera County\tH1\n59432\t30073\tDupuyer\tMT\tPondera County\tH1\n59416\t30073\tBrady\tMT\tPondera County\tH1\n59448\t30073\tHeart butte\tMT\tPondera County\tH1\n59486\t30073\tValier\tMT\tPondera County\tH1\n59314\t30075\tBiddle\tMT\tPowder River County\tH1\n59345\t30075\tPowderville\tMT\tPowder River County\tH1\n59317\t30075\tBroadus\tMT\tPowder River County\tH1\n59062\t30075\tOtter\tMT\tPowder River County\tH1\n59343\t30075\tOlive\tMT\tPowder River County\tH1\n59351\t30075\tVolborg\tMT\tPowder River County\tH1\n59854\t30077\tOvando\tMT\tPowell County\tH1\n59733\t30077\tGold creek\tMT\tPowell County\tH1\n59711\t30077\tAnaconda\tMT\tPowell County\tH1\n59843\t30077\tHelmville\tMT\tPowell County\tH1\n59713\t30077\tAvon\tMT\tPowell County\tH1\n59731\t30077\tGarrison\tMT\tPowell County\tH1\n59722\t30077\tDeer lodge\tMT\tPowell County\tH1\n59832\t30077\tDrummond\tMT\tPowell County\tH1\n59728\t30077\tElliston\tMT\tPowell County\tH1\n59339\t30079\tLindsay\tMT\tPrairie County\tH1\n59330\t30079\tGlendive\tMT\tPrairie County\tH1\n59349\t30079\tTerry\tMT\tPrairie County\tH1\n59336\t30079\tIsmay\tMT\tPrairie County\tH1\n59341\t30079\tMildred\tMT\tPrairie County\tH1\n59214\t30079\tBrockway\tMT\tPrairie County\tH1\n59326\t30079\tFallon\tMT\tPrairie County\tH1\n59840\t30081\tHamilton\tMT\tRavalli County\tH1\n59841\t30081\tPinesdale\tMT\tRavalli County\tH1\n59833\t30081\tFlorence\tMT\tRavalli County\tH1\n59870\t30081\tStevensville\tMT\tRavalli County\tH1\n59871\t30081\tSula\tMT\tRavalli County\tH1\n59875\t30081\tVictor\tMT\tRavalli County\tH1\n59829\t30081\tDarby\tMT\tRavalli County\tH1\n59835\t30081\tGrantsdale\tMT\tRavalli County\tH1\n59828\t30081\tCorvallis\tMT\tRavalli County\tH1\n59827\t30081\tConner\tMT\tRavalli County\tH1\n59221\t30083\tFairview\tMT\tRichland County\tH1\n59259\t30083\tRichey\tMT\tRichland County\tH1\n59270\t30083\tSidney\tMT\tRichland County\tH1\n59213\t30083\tBrockton\tMT\tRichland County\tH1\n59255\t30083\tPoplar\tMT\tRichland County\tH1\n59218\t30083\tCulbertson\tMT\tRichland County\tH1\n59243\t30083\tLambert\tMT\tRichland County\tH1\n59262\t30083\tSavage\tMT\tRichland County\tH1\n59217\t30083\tCrane\tMT\tRichland County\tH1\n59212\t30085\tBainville\tMT\tRoosevelt County\tH1\n59201\t30085\tWolf point\tMT\tRoosevelt County\tH1\n59213\t30085\tBrockton\tMT\tRoosevelt County\tH1\n59255\t30085\tPoplar\tMT\tRoosevelt County\tH1\n59218\t30085\tCulbertson\tMT\tRoosevelt County\tH1\n59242\t30085\tHomestead\tMT\tRoosevelt County\tH1\n59258\t30085\tReserve\tMT\tRoosevelt County\tH1\n59226\t30085\tFroid\tMT\tRoosevelt County\tH1\n59323\t30087\tColstrip\tMT\tRosebud County\tH1\n59003\t30087\tAshland\tMT\tRosebud County\tH1\n59347\t30087\tRosebud\tMT\tRosebud County\tH1\n59333\t30087\tHathaway\tMT\tRosebud County\tH1\n59312\t30087\tAngela\tMT\tRosebud County\tH1\n59327\t30087\tForsyth\tMT\tRosebud County\tH1\n59043\t30087\tLame deer\tMT\tRosebud County\tH1\n59012\t30087\tBirney\tMT\tRosebud County\tH1\n59039\t30087\tIngomar\tMT\tRosebud County\tH1\n59004\t30087\tAshland\tMT\tRosebud County\tH1\n59083\t30087\tSumatra\tMT\tRosebud County\tH1\n59821\t30089\tArlee\tMT\tSanders County\tH1\n59845\t30089\tHot springs\tMT\tSanders County\tH1\n59831\t30089\tDixon\tMT\tSanders County\tH1\n59856\t30089\tParadise\tMT\tSanders County\tH1\n59853\t30089\tNoxon\tMT\tSanders County\tH1\n59874\t30089\tTrout creek\tMT\tSanders County\tH1\n59873\t30089\tThompson falls\tMT\tSanders County\tH1\n59844\t30089\tHeron\tMT\tSanders County\tH1\n59859\t30089\tPlains\tMT\tSanders County\tH1\n59866\t30089\tSaint regis\tMT\tSanders County\tH1\n59848\t30089\tLonepine\tMT\tSanders County\tH1\n59252\t30091\tOutlook\tMT\tSheridan County\tH1\n59275\t30091\tWestby\tMT\tSheridan County\tH1\n59254\t30091\tPlentywood\tMT\tSheridan County\tH1\n59256\t30091\tRaymond\tMT\tSheridan County\tH1\n59219\t30091\tDagmar\tMT\tSheridan County\tH1\n59211\t30091\tAntelope\tMT\tSheridan County\tH1\n59247\t30091\tMedicine lake\tMT\tSheridan County\tH1\n59242\t30091\tHomestead\tMT\tSheridan County\tH1\n59258\t30091\tReserve\tMT\tSheridan County\tH1\n59257\t30091\tRedstone\tMT\tSheridan County\tH1\n59701\t30093\tButte\tMT\tSilver Bow County\tH6\n59711\t30093\tAnaconda\tMT\tSilver Bow County\tH6\n59759\t30093\tWhitehall\tMT\tSilver Bow County\tH6\n59703\t30093\tButte\tMT\tSilver Bow County\tH6\n59743\t30093\tMelrose\tMT\tSilver Bow County\tH6\n59762\t30093\tWise river\tMT\tSilver Bow County\tH6\n59702\t30093\tButte\tMT\tSilver Bow County\tH6\n59727\t30093\tDivide\tMT\tSilver Bow County\tH6\n59750\t30093\tButte\tMT\tSilver Bow County\tH6\n59748\t30093\tRamsay\tMT\tSilver Bow County\tH6\n59011\t30095\tBig timber\tMT\tStillwater County\tH1\n59057\t30095\tMolt\tMT\tStillwater County\tH1\n59074\t30095\tRyegate\tMT\tStillwater County\tH1\n59044\t30095\tLaurel\tMT\tStillwater County\tH1\n59069\t30095\tReed point\tMT\tStillwater County\tH1\n59019\t30095\tColumbus\tMT\tStillwater County\tH1\n59001\t30095\tAbsarokee\tMT\tStillwater County\tH1\n59063\t30095\tPark city\tMT\tStillwater County\tH1\n59028\t30095\tFishtail\tMT\tStillwater County\tH1\n59067\t30095\tRapelje\tMT\tStillwater County\tH1\n59046\t30095\tLavina\tMT\tStillwater County\tH1\n59070\t30095\tRoberts\tMT\tStillwater County\tH1\n59061\t30095\tNye\tMT\tStillwater County\tH1\n59015\t30095\tBroadview\tMT\tStillwater County\tH1\n59011\t30097\tBig timber\tMT\tSweet Grass County\tH1\n59055\t30097\tMelville\tMT\tSweet Grass County\tH1\n59069\t30097\tReed point\tMT\tSweet Grass County\tH1\n59033\t30097\tGreycliff\tMT\tSweet Grass County\tH1\n59070\t30097\tRoberts\tMT\tSweet Grass County\tH1\n59052\t30097\tMc leod\tMT\tSweet Grass County\tH1\n59082\t30097\tSpringdale\tMT\tSweet Grass County\tH1\n59422\t30099\tChoteau\tMT\tTeton County\tH1\n59468\t30099\tPower\tMT\tTeton County\tH1\n59467\t30099\tPendroy\tMT\tTeton County\tH1\n59425\t30099\tConrad\tMT\tTeton County\tH1\n59487\t30099\tVaughn\tMT\tTeton County\tH1\n59436\t30099\tFairfield\tMT\tTeton County\tH1\n59433\t30099\tDutton\tMT\tTeton County\tH1\n59443\t30099\tFort shaw\tMT\tTeton County\tH1\n59419\t30099\tBynum\tMT\tTeton County\tH1\n59466\t30101\tOilmont\tMT\tToole County\tH1\n59545\t30101\tWhitlash\tMT\tToole County\tH1\n59425\t30101\tConrad\tMT\tToole County\tH1\n59454\t30101\tKevin\tMT\tToole County\tH1\n59484\t30101\tSweet grass\tMT\tToole County\tH1\n59456\t30101\tLedger\tMT\tToole County\tH1\n59444\t30101\tGalata\tMT\tToole County\tH1\n59482\t30101\tSunburst\tMT\tToole County\tH1\n59427\t30101\tCut bank\tMT\tToole County\tH1\n59474\t30101\tShelby\tMT\tToole County\tH1\n59435\t30101\tEthridge\tMT\tToole County\tH1\n59461\t30101\tLothair\tMT\tToole County\tH1\n59038\t30103\tHysham\tMT\tTreasure County\tH1\n59010\t30103\tBighorn\tMT\tTreasure County\tH1\n59327\t30103\tForsyth\tMT\tTreasure County\tH1\n59076\t30103\tSanders\tMT\tTreasure County\tH1\n59248\t30105\tNashua\tMT\tValley County\tH1\n59273\t30105\tVandalia\tMT\tValley County\tH1\n59244\t30105\tLarslan\tMT\tValley County\tH1\n59253\t30105\tPeerless\tMT\tValley County\tH1\n59223\t30105\tFort peck\tMT\tValley County\tH1\n59250\t30105\tOpheim\tMT\tValley County\tH1\n59201\t30105\tWolf point\tMT\tValley County\tH1\n59261\t30105\tSaco\tMT\tValley County\tH1\n59260\t30105\tRichland\tMT\tValley County\tH1\n59240\t30105\tGlentana\tMT\tValley County\tH1\n59231\t30105\tSaint marie\tMT\tValley County\tH1\n59230\t30105\tGlasgow\tMT\tValley County\tH1\n59241\t30105\tHinsdale\tMT\tValley County\tH1\n59225\t30105\tFrazer\tMT\tValley County\tH1\n59078\t30107\tShawmut\tMT\tWheatland County\tH1\n59074\t30107\tRyegate\tMT\tWheatland County\tH1\n59036\t30107\tHarlowton\tMT\tWheatland County\tH1\n59453\t30107\tJudith gap\tMT\tWheatland County\tH1\n59085\t30107\tTwo dot\tMT\tWheatland County\tH1\n59353\t30109\tWibaux\tMT\tWibaux County\tH1\n59101\t30111\tBillings\tMT\tYellowstone County\tH1\n59057\t30111\tMolt\tMT\tYellowstone County\tH1\n59044\t30111\tLaurel\tMT\tYellowstone County\tH1\n59107\t30111\tBillings\tMT\tYellowstone County\tH1\n59103\t30111\tBillings\tMT\tYellowstone County\tH1\n59041\t30111\tJoliet\tMT\tYellowstone County\tH1\n59079\t30111\tShepherd\tMT\tYellowstone County\tH1\n59064\t30111\tPompeys pillar\tMT\tYellowstone County\tH1\n59006\t30111\tBallantine\tMT\tYellowstone County\tH1\n59088\t30111\tWorden\tMT\tYellowstone County\tH1\n59063\t30111\tPark city\tMT\tYellowstone County\tH1\n59106\t30111\tBillings\tMT\tYellowstone County\tH1\n59108\t30111\tBillings\tMT\tYellowstone County\tH1\n59002\t30111\tActon\tMT\tYellowstone County\tH1\n59111\t30111\tBillings\tMT\tYellowstone County\tH1\n59102\t30111\tBillings\tMT\tYellowstone County\tH1\n59105\t30111\tBillings\tMT\tYellowstone County\tH1\n59104\t30111\tBillings\tMT\tYellowstone County\tH1\n59024\t30111\tCuster\tMT\tYellowstone County\tH1\n59037\t30111\tHuntley\tMT\tYellowstone County\tH1\n59015\t30111\tBroadview\tMT\tYellowstone County\tH1\n68955\t31001\tJuniata\tNE\tAdams County\tH1\n68956\t31001\tKenesaw\tNE\tAdams County\tH1\n68945\t31001\tHeartwell\tNE\tAdams County\tH1\n68957\t31001\tLawrence\tNE\tAdams County\tH1\n68973\t31001\tRoseland\tNE\tAdams County\tH1\n68883\t31001\tWood river\tNE\tAdams County\tH1\n68928\t31001\tBladen\tNE\tAdams County\tH1\n68925\t31001\tAyr\tNE\tAdams County\tH1\n68930\t31001\tBlue hill\tNE\tAdams County\tH1\n68950\t31001\tHolstein\tNE\tAdams County\tH1\n68902\t31001\tHastings\tNE\tAdams County\tH1\n68901\t31001\tHastings\tNE\tAdams County\tH1\n68941\t31001\tGlenvil\tNE\tAdams County\tH1\n68932\t31001\tCampbell\tNE\tAdams County\tH1\n68980\t31001\tTrumbull\tNE\tAdams County\tH1\n68781\t31003\tTilden\tNE\tAntelope County\tH1\n68769\t31003\tPlainview\tNE\tAntelope County\tH1\n68652\t31003\tPetersburg\tNE\tAntelope County\tH1\n68720\t31003\tBrunswick\tNE\tAntelope County\tH1\n68726\t
